vi "AH2500.BIAS.vi"(7 "error in (no error)":errorcluster, 9 "DC Bias":T1(ring), 10 "VISA resource name":refnum<visa-resource-name>) -> (0 "error out":errorcluster, 1 "Send":string, 2 "Result":string, 3 "VISA resource name out":refnum<visa-resource-name>)   [LabVIEW 2019, in "Inst.AH2500.lvclass"]
uses:
  Inst.AH2500.lvclass
panel:
  # "DC bias enable setting"
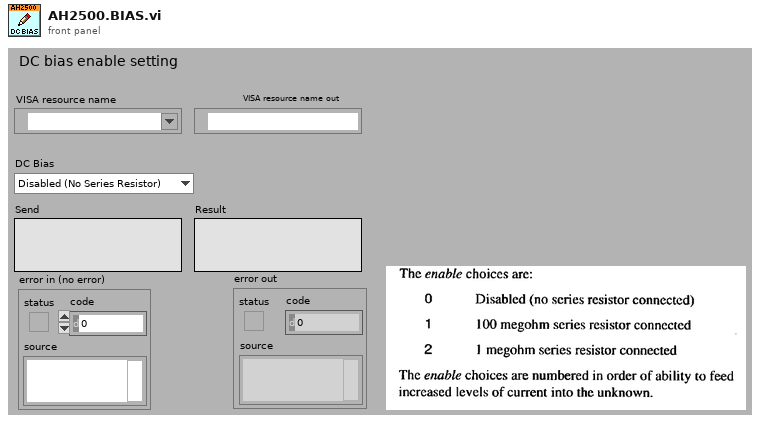
[diagram p1: front panel]
types:
  T1 = enum16{"Disabled (No Series Resistor)", "100 MOhm Series Resistor", "1 MOhm Series Resistor"}
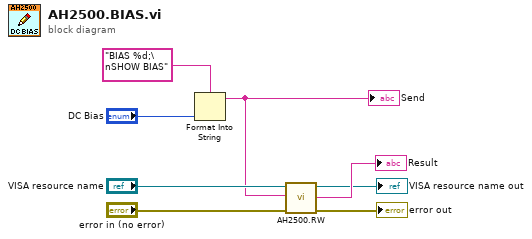
[diagram p0: block diagram]
diagram:
  n1 = Format Into String(format string="BIAS %d;\nSHOW BIAS", "DC Bias") -> (resulting string=w5:string)  [unwired: 2 in, 1 out]
  "Send" <- w5
  n2 = call "AH2500.RW.vi"("error in (no error)"="error in (no error)", "write buffer"=w5, "VISA Refnum in"="VISA resource name") -> ("error out"=→"error out":errorcluster, "read buffer"=→"Result":string, "VISA Refnum out"=→"VISA resource name out":refnum<visa-resource-name>)  [unwired: 6 in]
